vi "Filter string array.vi"(2 "Elements to Match":string[](array[string]), 3 "Array to Search":string[](array[string])) -> (0 "Remaining Elements":string[](array[string]), 1 "Found Elements":string[](array[string]))   [LabVIEW 2020, in "verticalDistribution.lvlib"]
uses:
  <vilib>/Utility/vertDist/verticalDistribution.lvlib
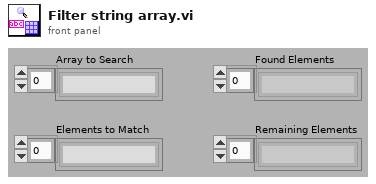
[diagram p1: front panel]
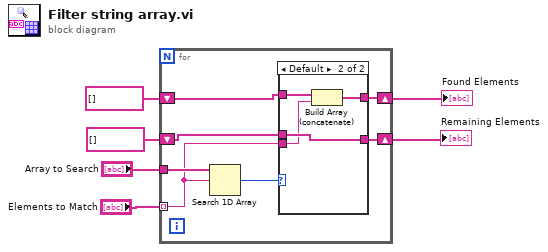
[diagram p0: block diagram]
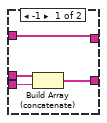
[diagram p2: hidden frame]
diagram:
  n1 = for {
    tunnel: "Array to Search" -> [w13]
    tunnel: "Elements to Match" -> [w12] mode=indexing
    shift-right: [w11] -> w4
    shift-left: string[] [] -> [w10]
    shift-right: [w8] -> w6
    shift-left: string[] [] -> [w9]
    n2 = Search 1D Array(1D array=w13, element=w12) -> (index of element=w7:i32)  [unwired: 1 out]
    n3 = case shown="Default" w7 {
      tunnel: w12 -> [w15 w19]
      tunnel: [w17 w21] -> w11
      tunnel: w10 -> [w16 w21]
      tunnel: w9 -> [w14 w20]
      tunnel: [w14 w18] -> w8
      frame -1 {
        n4 = Build Array (concatenate)(w16, w15) -> (w17:string[])
      }
      frame Default {
        n5 = Build Array (concatenate)(w20, w19) -> (w18:string[])
      }
    }
  }
  "Found Elements" <- w6
  "Remaining Elements" <- w4
